vi "ReadFilesInFolder.vi"(7 "Current File In":i32, 8 "error in (no error)":errorcluster, 9 "Read entire Folder":bool, 10 "FolderPath":path, 11 "Current File Path":path) -> (0 "error out":errorcluster, 1 "Current File Path":path, 2 "Current File Out":i32, 3 "filenames":string[](array[string]))   [LabVIEW 2020]
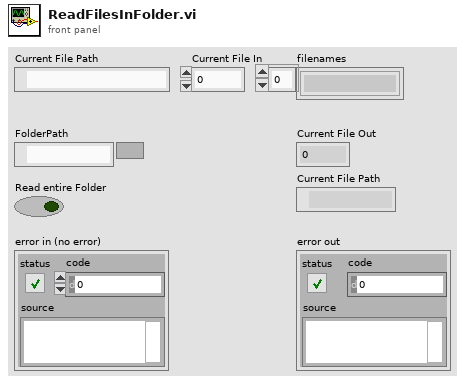
[diagram p1: front panel]
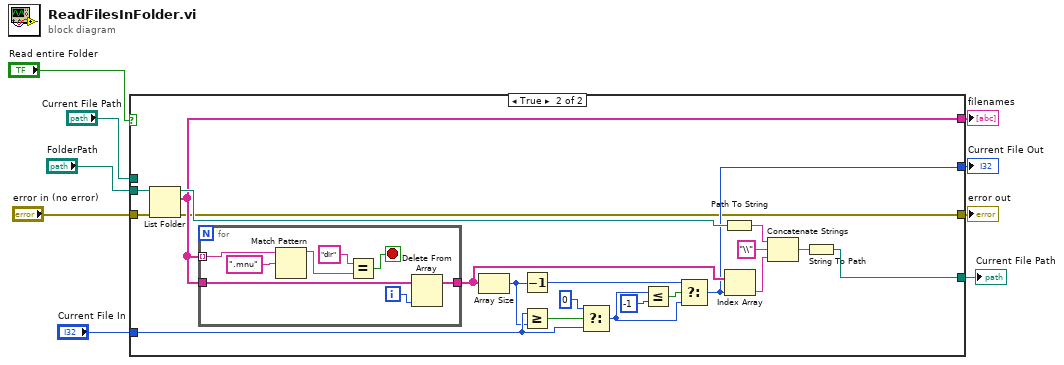
[diagram p0: block diagram]
diagram:
  n1 = case shown="True" "Read entire Folder" {
    tunnel: "error in (no error)" -> [w11 w28]
    tunnel: "Current File In" -> [w12 w26]
    tunnel: [w12 w17] -> w5
    tunnel: [w11 w14] -> w6
    tunnel: "FolderPath" -> [_ w16]
    tunnel: [_ w15] -> w9
    tunnel: "Current File Path" -> [w10 _]
    tunnel: [w10 w13] -> w1
    frame False {
    }
    frame True {
      n2 = List Folder(path=w16, error in=w28) -> (path out=w32:path, filenames=w15:string[], error out=w14:errorcluster)  [unwired: 2 in, 1 out]
      n3 = for {
        tunnel: w15 -> [w40] mode=indexing
        tunnel: w15 -> [w37]
        tunnel: [w33] -> w23
        i -> [w38]
        stop <- w34 stop-if-true
        n4 = Match Pattern(string=w40, regular expression=".mnu" ("string")) -> (before substring=w35:string)  [unwired: 1 in, 3 out]
        n5 = Equal?(x="dir" ("string"), y=w35) -> (x = y?=w34:bool)
        n6 = Delete From Array(array=w37, index=w38) -> (array with subset deleted=w33:string[])  [unwired: 1 in, 1 out]
      }
      n7 = Array Size(array=w23) -> (size(s)=w20:i32)
      n8 = Decrement(x=w20) -> (x-1=w19:i32)
      n9 = Greater Or Equal?(x=w26, y=w20) -> (x >= y?=w27:bool)
      n10 = Select(t=0, s=w27, f=w26) -> (s? t:f=w18:i32)
      n11 = Less Or Equal?(x=w18, y=-1) -> (x <= y?=w21:bool)
      n12 = Select(t=w19, s=w21, f=w18) -> (s? t:f=w17:i32)
      n13 = Path To String(path=w32) -> (string=w31:string)
      n14 = Index Array(array=w23, index=w17) -> (element=w24:string)
      n15 = Concatenate Strings(w31, "\\" ("string"), w24) -> (w30:string)
      n16 = String To Path(string=w30) -> (path=w13:path)
    }
  }
  "filenames" <- w9
  "error out" <- w6
  "Current File Out" <- w5
  "Current File Path" <- w1
